vi "App Name.vi"(11 "App in":refnum<class "App.lvclass">) -> (2 "App Name":string)   [LabVIEW 2020, in "Volatus.lvlib" / "App.lvclass"]
uses:
  App.lvclass
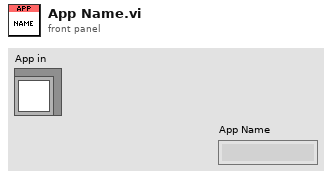
[diagram p1: front panel]
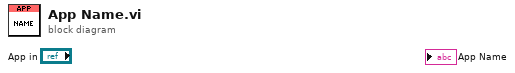
[diagram p0: block diagram]
diagram:
